vi "Verify Digital Waveform in LV.vi"(2 "Y":digitaldata, 3 "dt":dbl, 4 "t0":timestamp, 5 "digital waveform":digitalwaveform(waveform)={"t0"=timestamp(0 s since 1904-01-01), "dt"=0.0, "Y"={"transitions"=[], "data"=[]}, "error"={"status"=FALSE, "code"=37421928, "source"=""}}) -> (0 "Components Equal":bool, 1 "digital waveform out":digitalwaveform(waveform)={"t0"=timestamp(0 s since 1904-01-01), "dt"=0.0, "Y"={"transitions"=[], "data"=[]}, "error"={"status"=FALSE, "code"=37421928, "source"=""}})   [LabVIEW 2012]
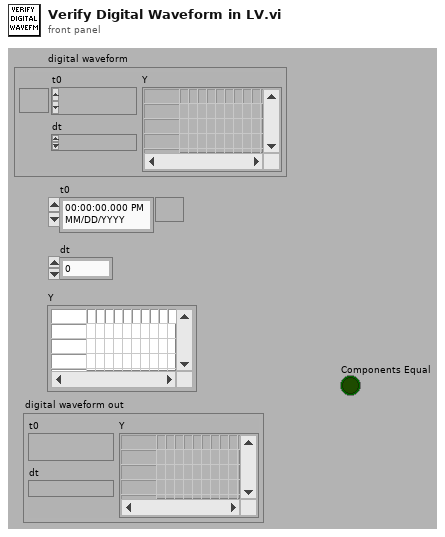
[diagram p1: front panel]
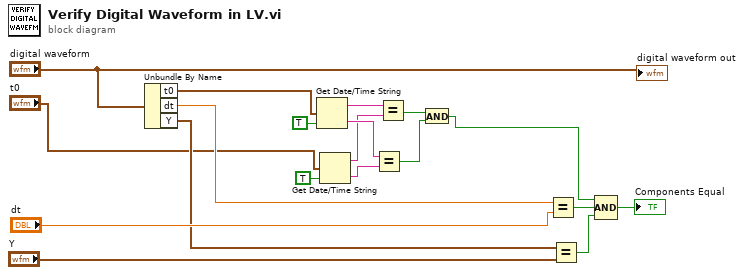
[diagram p0: block diagram]
diagram:
  n1 = Unbundle By Name("digital waveform") -> ("t0"=w9:timestamp, "dt"=w18:dbl, "Y"=w16:digitaldata)
  n2 = Get Date/Time String(seconds (now)=w9, want seconds? (F)=TRUE) -> (date string=w4:string, time string=w7:string)  [unwired: 1 in]
  n3 = Get Date/Time String(seconds (now)="t0", want seconds? (F)=TRUE) -> (date string=w5:string, time string=w6:string)  [unwired: 1 in]
  n4 = Equal?(x=w7, y=w6) -> (x = y?=w3:bool)
  n5 = Equal?(x=w4, y=w5) -> (x = y?=w2:bool)
  n6 = And(x=w2, y=w3) -> (x .and. y?=w1:bool)
  n7 = Equal?(x=w18, y="dt") -> (x = y?=w14:bool)
  n8 = Equal?(x=w16, y="Y") -> (x = y?=w13:bool)
  n9 = Compound Arithmetic op=AND(w1, w14, w13) -> (→"Components Equal":bool)
  "digital waveform out" <- "digital waveform"
